vi "sub_SDR_demod_QAM4.vi"(11 "Input Symbols":cdb[](array[numeric])) -> (3 "Demodulated data":bool[](array[boolean]))   [LabVIEW 2012]
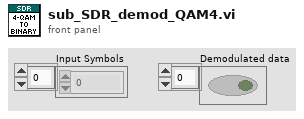
[diagram p1: front panel]
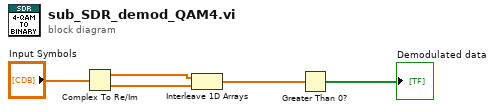
[diagram p0: block diagram]
diagram:
  n1 = Complex To Re/Im(x + iy="Input Symbols") -> (x=w2:dbl[], y=w3:dbl[])
  n2 = Interleave 1D Arrays "Interleave 1D Arrays"(w2, w3) -> (w1:dbl[])
  n3 = Greater Than 0?(x=w1) -> (x > 0?=→"Demodulated data":bool[])
